vi "Read Config.vi"(8 "error in (no error)":errorcluster, 10 "Resource In":variant, 11 "Analyze Parameter Base in":refnum<class "Analyze Parameter Base.lvclass">) -> (0 "error out":errorcluster, 2 "Resource Out":variant, 3 "Analyze Parameter Base out":refnum<class "Analyze Parameter Base.lvclass">)   [LabVIEW 2020, in "Analyze Parameter Base.lvclass"]
uses:
  Analyze Parameter Base.lvclass
  Analyze Parameter Base.lvclass/Analyze Parameter Base.ctl
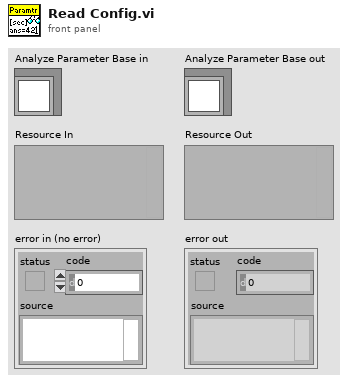
[diagram p1: front panel]
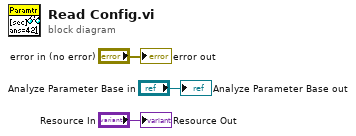
[diagram p0: block diagram]
diagram:
  "error out" <- "error in (no error)"
  "Analyze Parameter Base out" <- "Analyze Parameter Base in"
  "Resource Out" <- "Resource In"
